vi "Setup UI.vi"(8 "error in (no error)":errorcluster, 10 "Set UI to input? (F)":bool, 11 "DAQmx Analog in":refnum<class "DAQmx Analog.lvclass">) -> (0 "error out":errorcluster, 3 "DAQmx Analog out":refnum<class "DAQmx Analog.lvclass">)   [LabVIEW 2012, in "DAQmx Analog.lvclass"]
doc: "Setup UI constructs an object -- populates its member data -- from a front panel the user can see. The VI should be as simple as possible so that a UI loop can poll it continuously for updates. \n\nThe VI is designed to be used as a subPanel within another VI. Wire true to \"Set UI to input\" only on the first call, just after inserting this VI into a subPanel, to populate its controls with the class's current values.\n\nSetup UI is distinct from the class constructor. Class constructors are not polymorphic, yet configure dialogs need to configure objects without knowing their type -- and polymorphism is the necessary solution. Thus, Setup UI is a polymorphic class constructor. This continously polled \"Setup UI\" concept is a kludge: a better idea would be an XControl, but those require a steeper learning curve."
uses:
  DAQmx Analog.lvclass
  Utility Classes/Readable/Readable.lvclass
panel:
  in  "Analog input #":u8
  # "DAQmx Analog Setup"
  # "This Setup pane does nothing right now."
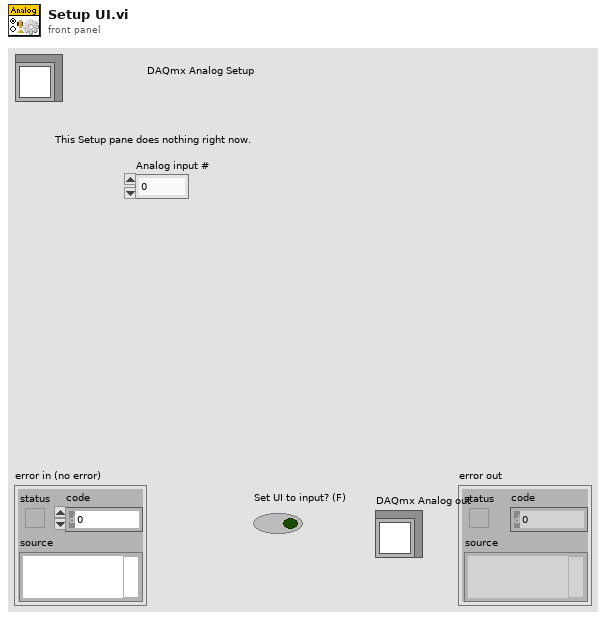
[diagram p1: front panel]
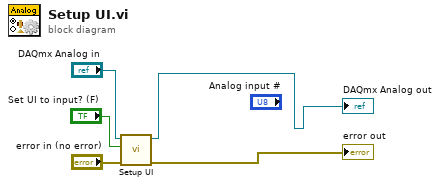
[diagram p0: block diagram]
diagram:
  n1 = call-parent "Setup UI.vi"("error in (no error)"="error in (no error)", "Set UI to input? (F)"="Set UI to input? (F)", "Instrument in"="DAQmx Analog in") -> ("error out"=→"error out":errorcluster, "Instrument out"=→"DAQmx Analog out":refnum<class "DAQmx Analog.lvclass">)  [unwired: 7 out]
